vi "2D_Array_to_Waveform.vi"(1 "Y":dbl[](array[numeric]) format="%_6g", 2 "X":dbl[](array[numeric]), 3 "Nº de amostras":i32=128) -> (0 "output waveform":waveform(dbl))   [LabVIEW 2018]
doc: "Esse VI converte um sinal de duas dimensões (composto por um vetor x e um vetor y) em um waveform. Caso o vetor não tenha um intervalo de tempo homogêneo, a função inerpola o sinal, gerando uma waveform um novo intervalo de tempo fixo."
uses:
  <vilib>/Analysis/1siggen.llb/Ramp Pattern by Samples.vi
  <vilib>/Analysis/NI_AALBase.lvlib
  <vilib>/gmath/NI_Gmath.lvlib
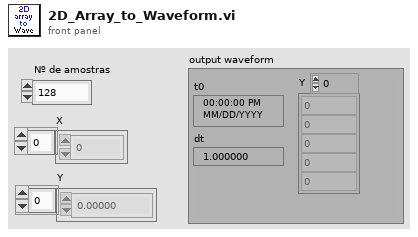
[diagram p1: front panel]
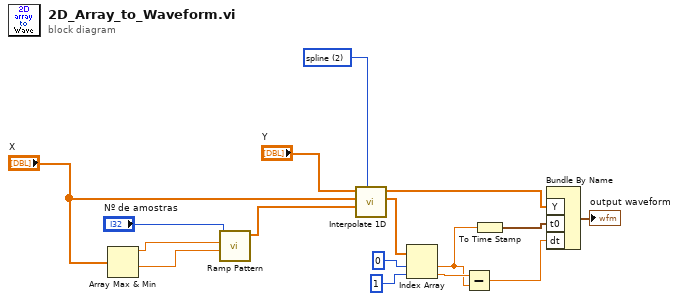
[diagram p0: block diagram]
diagram:
  w15 = 2 items=["nearest", "linear", "spline", "cubic Hermite", "Lagrange"] ("method")
  n1 = Array Max & Min(array="X") -> (max value=w2:dbl, min value=w1:dbl)  [unwired: 2 out]
  n2 = call-poly <vilib>:"Ramp Pattern.vi"("start"=w1, "end"=w2, "samples"="Nº de amostras") -> ("Ramp Pattern"=w12:dbl[])  [unwired: 7 in, 1 out]
  n3 = call <vilib>:"Interpolate 1D.vi"("method"=w15, "xi"=w12, "X"="X", "Y"="Y") -> ("xi used"=w10:dbl[], "yi"=w11:dbl[])  [unwired: 5 in, 1 out]
  n4 = Index Array "Index Array"(array=w10, index #1=0 ("index"), index #2=1 ("index")) -> (element #1=w7:dbl, element #2=w9:dbl)
  n5 = Subtract(x=w9, y=w7) -> (x-y=w6:dbl)
  n6 = To Time Stamp(1:w7) -> (0:w8:timestamp)
  n7 = Bundle By Name("Y"=w11, "t0"=w8, "dt"=w6) -> (→"output waveform":waveform(dbl))  [unwired: 1 in]
